vi "Device Resources.vi"(8 "error in (no error)":errorcluster, 11 "FirmwareComms in":refnum<class "VisaComms.lvclass">) -> (0 "error out":errorcluster, 2 "Resource Info":T1, 3 "FirmwareComms out":refnum<class "VisaComms.lvclass">)   [LabVIEW 2020, in "CTI.lvlib" / "VisaComms.lvclass"]
uses:
  VisaComms.lvclass
  Resource Info.ctl
  CTI.lvlib
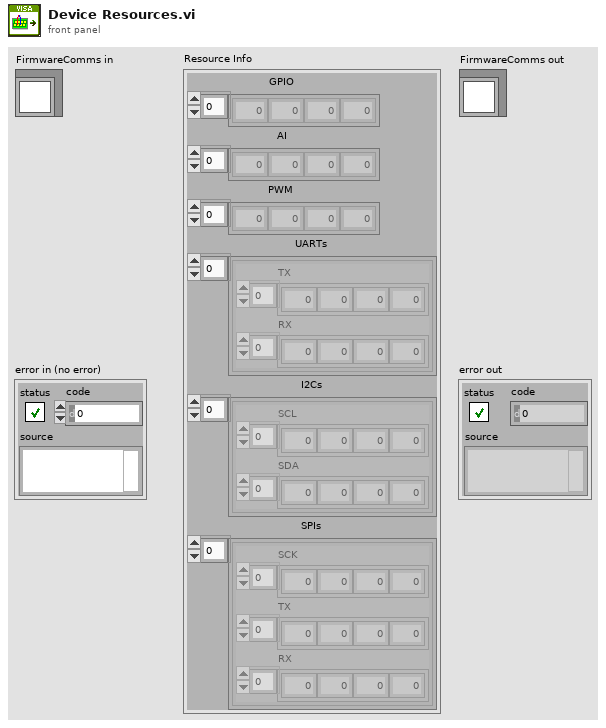
[diagram p1: front panel]
types:
  T1 = typedef "CTI.lvlib/Resource Info.ctl" = cluster{"GPIO":u8[], "AI":u8[], "PWM":u8[], "UARTs":cluster{"TX":u8[], "RX":u8[]}[], "I2Cs":cluster{"SCL":u8[], "SDA":u8[]}[], "SPIs":cluster{"SCK":u8[], "TX":u8[], "RX":u8[]}[]}
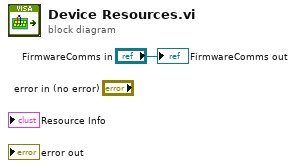
[diagram p0: block diagram]
diagram:
  "FirmwareComms out" <- "FirmwareComms in"
